vi "Jaden_Payton_Lab7_Systems_Correct.vi"() -> ()   [LabVIEW 2021]
uses:
  <vilib>/Platform/TimedLoop/XDataNode/timing_clust.ctl
  <vilib>/Platform/TimedLoop/XDataNode/nitl_modes.ctl
  <vilib>/Platform/TimedLoop/XDataNode/wakeup.ctl
  <vilib>/DAQmx/read.llb/DAQmx Read (Analog 2D DBL NChan NSamp).vi
  <vilib>/DAQmx/create/channels.llb/DAQmx Create Channel (AI-Voltage-Basic).vi
  <vilib>/DAQmx/configure/timing.llb/DAQmx Timing (Sample Clock).vi
  <vilib>/DAQmx/miscellaneous.llb/DAQmx Fill In Error Info.vi
  <vilib>/platform/TimedLoop/XDataNode/XDataNode.xnode
  <vilib>/Platform/TimedLoop/XDataNode/XDNodeRunTimeDep.lvlib
panel:
  out "SPO2":dbl
  out "Filtered IR LED":dbl(graph)
  out "Filtered Red LED":dbl(graph)
  in  "N 2":i32
  out "appended array 2":dbl[](array[numeric])
  out "IR LED":dbl[](graph)
  out "Red LED":dbl[](graph)
  in  "stop":bool
  in  "N":i32
  out "appended array":dbl[](array[numeric])
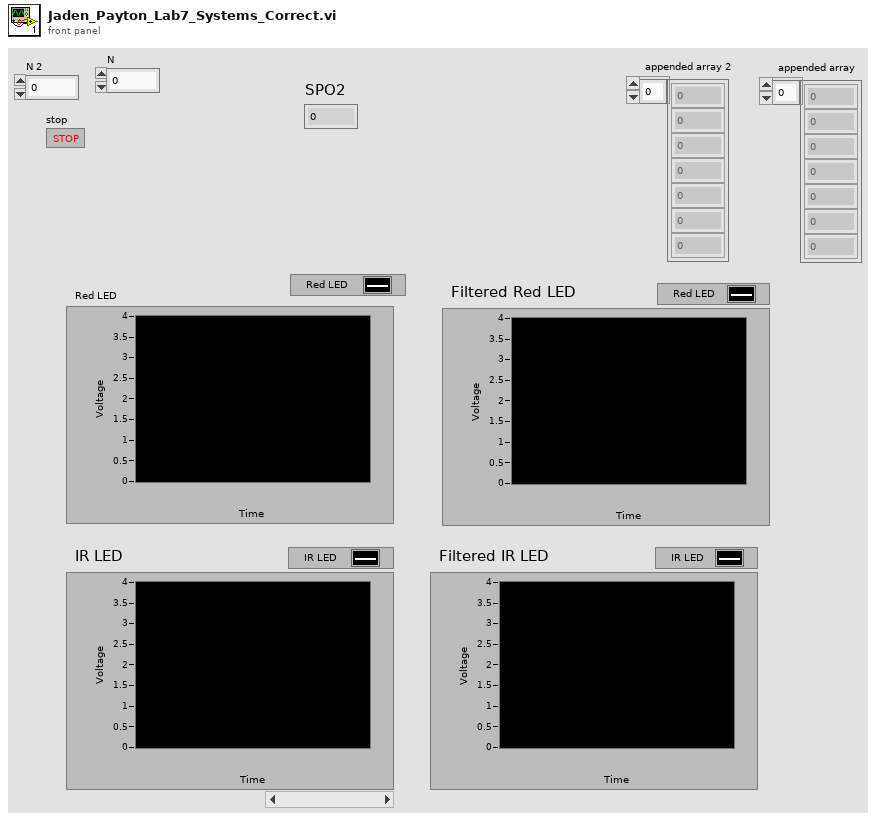
[diagram p1: front panel]
types:
  T1 = typedef "XDNodeRunTimeDep.lvlib/timing_clust.ctl" = cluster{"Expected End [f-1]":u64, "Actual End [f-1]":u64, "Finished Late? [f-1]":bool, "Expected End [i-1]":u64, "Actual End [i-1]":u64, "Finished Late? [i-1]":bool, "Expected Start [i]":u64, "Actual Start [i]":u64, "Expected Start [f]":u64, "Actual Start [f]":u64, "Source Name":string, "Structure Name":string, "Period":i64, "Deadline":i64, "Offset":i64, "Start":i64, "Priority":i32, "Timeout":i32, "Mode":T2, "Wakeup Reason":T3, "Error":errorcluster, "Source Type":string, "Secondary Source Type":string, "Global End Time":u64, "Global Start Time":u64, "Frame Duration":u64, "Iteration Duration":u64, "Assigned CPU":i32, "I/O Scan Engine Mode":u32}
  T2 = typedef "XDNodeRunTimeDep.lvlib/nitl_modes.ctl" = enum32{"No Change", "Process missed periods, maintain original phase", "Discard missed periods, maintain original phase", "Process missed periods, ignore original phase", "Discard missed periods, ignore original phase"}
  T3 = typedef "XDNodeRunTimeDep.lvlib/wakeup.ctl" = enum32{"Normal", "Aborted", "Asynchronous wakeup", "Timing source error", "Timed loop error", "Timeout"}
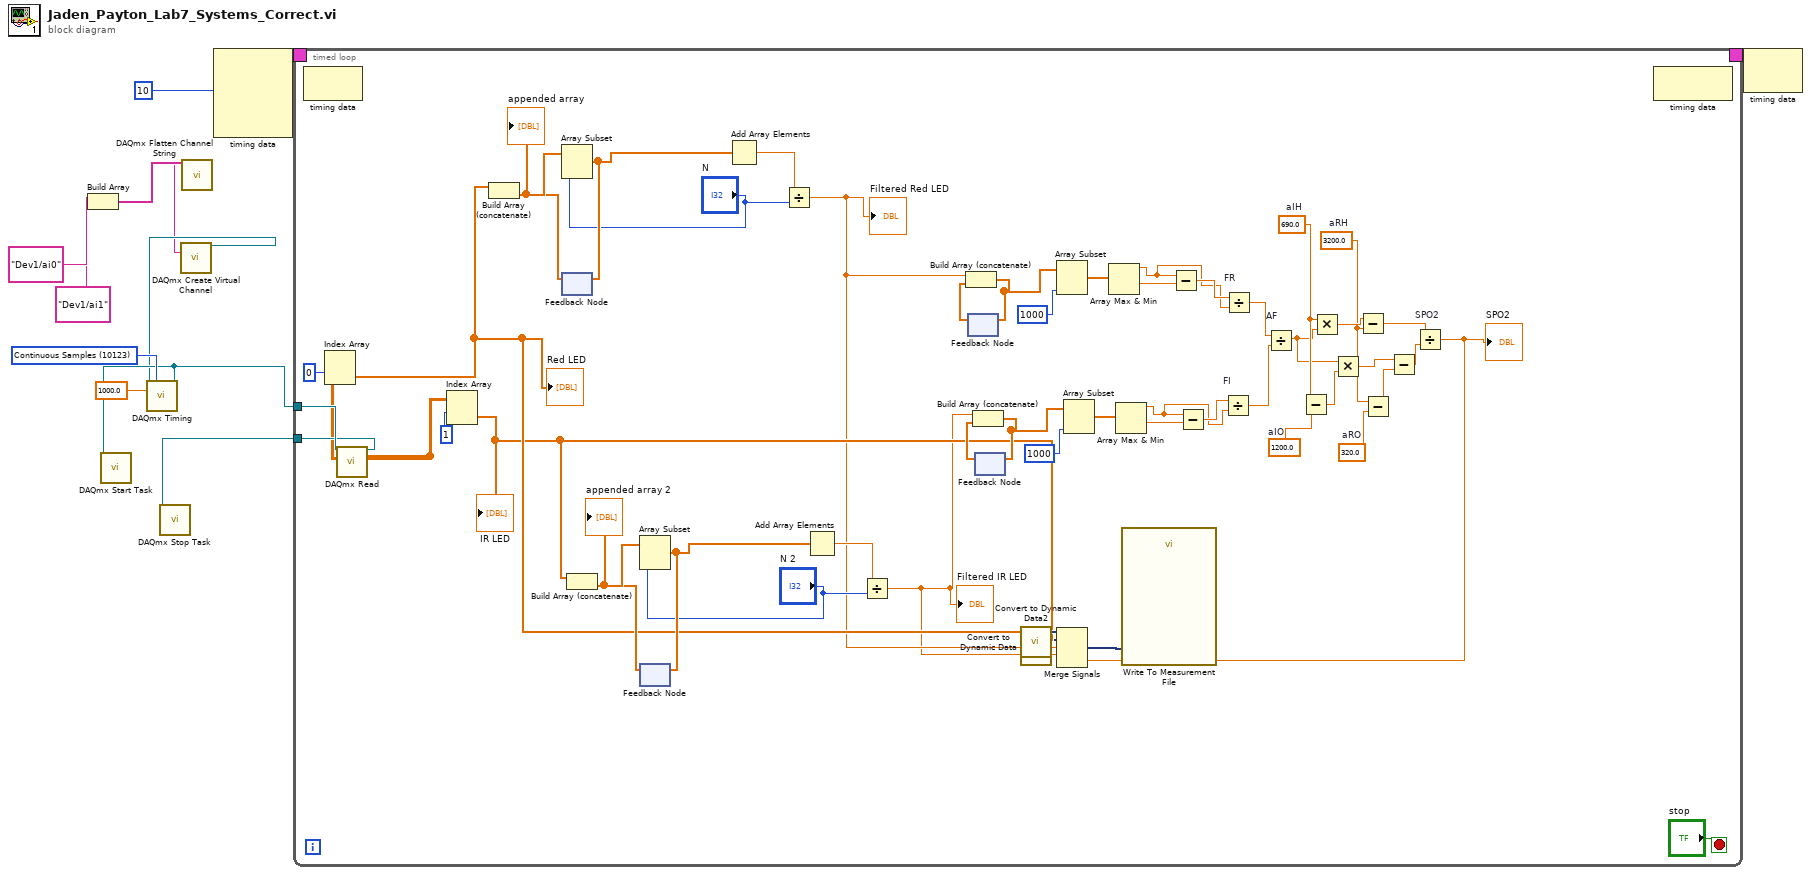
[diagram p0: block diagram]
diagram:
  w10 = 10123 items=["Finite Samples"=10178, "Continuous Samples"=10123, "Hardware Timed Single Point"=12522] ("sample mode")
  n1 = Build Array(tag "Dev1/ai0" ("physical channels"), tag "Dev1/ai1" ("physical channels")) -> (w2:tag[])
  n2 = call <vilib>:"DAQmx Flatten Channel String.vi"("names in"=w2) -> ("names out"=w1:string)  [unwired: 13 in, 1 out]
  n3 = call-poly <vilib>:"DAQmx Create Virtual Channel.vi"("physical channels"=w1) -> ("task out"=w5:refnum<k21>)  [unwired: 13 in, 1 out]
  n4 = call-poly <vilib>:"DAQmx Timing.vi"("task/channels in"=w5, "sample mode"=w10, "rate"=1000.0) -> ("task out"=w8:refnum<k21>)  [unwired: 11 in, 1 out]
  n5 = call <vilib>:"DAQmx Start Task.vi"("task/channels in"=w8) -> ()  [unwired: 13 in, 2 out]
  n6 = node-c288(i64 10 ("Period")) -> (w12:T1)  [unwired: 3 in]
  n7 = timed-loop {
    timing: w12 -> [_]
    timing-out: [_] -> w11
    tunnel: w8 -> [w57]
    tunnel: [w56] -> w7
    stop <- "stop" stop-if-true
    w27 = 320.0  # aRO
    w29 = 1200.0  # aIO
    w24 = 3200.0  # aRH
    w28 = 690.0  # aIH
    n8 = node-c288() -> ()  [unwired: 1 in, 1 out]
    n9 = call-poly <vilib>:"DAQmx Read.vi"("task/channels in"=w57) -> ("task out"=w56:refnum<k21>, "data"=w53:dbl[][])  [unwired: 12 in, 1 out]
    n10 = Index Array(array=w53, index (row)=0 ("index")) -> (element=w19:dbl[])  [unwired: 1 in]
    "Red LED" <- w19
    n11 = Index Array(array=w53, index (row)=1 ("index")) -> (element=w17:dbl[])  [unwired: 1 in]
    "IR LED" <- w17
    n12 = feedback #1() -> (w62:dbl[])  [unwired: 1 in]
    n13 = Build Array (concatenate)(w19, w62) -> (w63:dbl[])
    "appended array" <- w63
    n14 = Array Subset(array=w63, length="N") -> (w61:dbl[])  [unwired: 1 in]
    n15 = feedback-in #1(w61) -> ()
    n16 = feedback #2() -> (w51:dbl[])  [unwired: 1 in]
    n17 = Build Array (concatenate)(w17, w51) -> (w52:dbl[])
    "appended array 2" <- w52
    n18 = Array Subset(array=w52, length="N 2") -> (w50:dbl[])  [unwired: 1 in]
    n19 = feedback-in #2(w50) -> ()
    n20 = Add Array Elements(numeric array=w61) -> (sum=w60:dbl)
    n21 = Divide(x=w60, y="N") -> (x/y=w15:dbl)
    "Filtered Red LED" <- w15
    n22 = Add Array Elements(numeric array=w50) -> (sum=w49:dbl)
    n23 = Divide(x=w49, y="N 2") -> (x/y=w14:dbl)
    "Filtered IR LED" <- w14
    n24 = feedback #3() -> (w47:dbl[])  [unwired: 1 in]
    n25 = Build Array (concatenate)(w15, w47) -> (w46:dbl[])
    n26 = feedback-in #3(w46) -> ()
    n27 = feedback #4() -> (w40:dbl[])  [unwired: 1 in]
    n28 = Build Array (concatenate)(w14, w40) -> (w39:dbl[])
    n29 = feedback-in #4(w39) -> ()
    n30 = call "Convert to Dynamic Data"("Array"=w19) -> ("Dynamic Data Type"=w18:dynamicdata)  [unwired: 3 in]
    n31 = call "Convert to Dynamic Data2"("Array"=w17) -> ("Dynamic Data Type"=w16:dynamicdata)  [unwired: 3 in]
    n32 = Array Subset(array=w46, length=1000) -> (w44:dbl[])  [unwired: 1 in]
    n33 = Array Subset(array=w39, length=1000) -> (w37:dbl[])  [unwired: 1 in]
    n34 = Array Max & Min(array=w44) -> (max value=w41:dbl, min value=w43:dbl)  [unwired: 2 out]
    n35 = Array Max & Min(array=w37) -> (max value=w34:dbl, min value=w36:dbl)  [unwired: 2 out]
    n36 = Subtract(x=w41, y=w43) -> (x-y=w42:dbl)
    n37 = Subtract(x=w34, y=w36) -> (x-y=w35:dbl)
    n38 = Divide "FI"(x=w35, y=w34) -> (x/y=w32:dbl)
    n39 = Divide "FR"(x=w42, y=w41) -> (x/y=w33:dbl)
    n40 = Divide "AF"(x=w33, y=w32) -> (x/y=w26:dbl)
    n41 = Subtract(x=w28, y=w29) -> (x-y=w25:dbl)
    n42 = Multiply(x=w28, y=w26) -> (x*y=w31:dbl)
    n43 = Multiply(x=w26, y=w25) -> (x*y=w23:dbl)
    n44 = Subtract(x=w31, y=w24) -> (x-y=w30:dbl)
    n45 = Subtract(x=w24, y=w27) -> (x-y=w22:dbl)
    n46 = Subtract(x=w23, y=w22) -> (x-y=w21:dbl)
    n47 = Divide "SPO2"(x=w30, y=w21) -> (x/y=w13:dbl)
    "SPO2" <- w13
    n48 = Merge Signals(w18, w16, w15, w14, w13) -> (w20:dynamicdata)
    n49 = call "Write To Measurement File"("Signals"=w20) -> ()  [unwired: 16 in, 3 out]
    n50 = node-c288() -> ()  [unwired: 1 in, 1 out]
  }
  n51 = call <vilib>:"DAQmx Stop Task.vi"("task/channels in"=w7) -> ()  [unwired: 13 in, 2 out]
  n52 = node-c288(w11) -> ()  [unwired: 1 out]
